vi "Tools_System Memory Status.vi"(8 "error in (no error)":errorcluster) -> (0 "error out":errorcluster, 1 "Free memory (%)":dbl, 2 "Free memory (MB)":dbl, 3 "Total memory (MB)":dbl)   [LabVIEW 2013]
uses:
  kernel32.dll
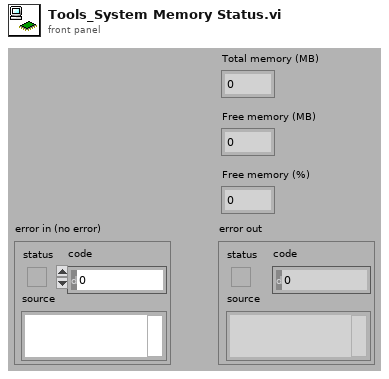
[diagram p1: front panel]
types:
  T1 = cluster{"dwLength":u32, "dwMemoryLoad":u32, "ullTotalPhys":u64, "ullAvailPhys":u64, "ullTotalPageFile":u64, "ullAvailPageFile":u64, "ullTotalVirtual":u64, "ullAvailVirtual":u64, "ullAvailExtendedVirtual":u64}
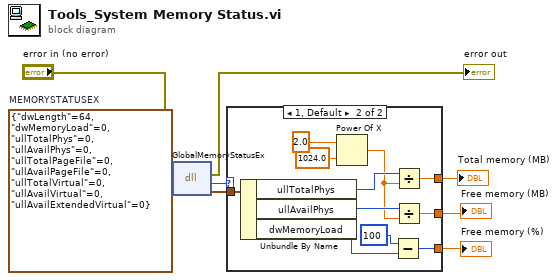
[diagram p0: block diagram]
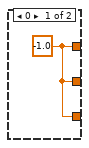
[diagram p2: hidden frame]
diagram:
  w3 = T1 {"dwLength"=64, "dwMemoryLoad"=0, "ullTotalPhys"=0, "ullAvailPhys"=0, "ullTotalPageFile"=0, "ullAvailPageFile"=0, "ullTotalVirtual"=0, "ullAvailVirtual"=0, "ullAvailExtendedVirtual"=0}  # MEMORYSTATUSEX
  n1 = dll-call lib="kernel32.dll" fn="GlobalMemoryStatusEx"(error in="error in (no error)", w3) -> (error out=→"error out":errorcluster, "return type"=w4:i32, w5:T1)  [unwired: 2 in, 1 out]
  n2 = case shown="1, Default" w4 {
    tunnel: w5 -> [_ w20]
    tunnel: [w9 w10] -> w8
    tunnel: [w9 w14] -> w6
    tunnel: [w9 w13] -> w7
    frame 0 {
      w9 = -1.0
    }
    frame 1, Default {
      n3 = Unbundle By Name(w20) -> ("ullTotalPhys"=w17:u64, "ullAvailPhys"=w16:u64, "dwMemoryLoad"=w11:u32)
      n4 = Power Of X(1:1024.0 ("x"), 2:2.0 ("y")) -> (0:w15:dbl)
      n5 = Subtract(x=u32 100, y=w11) -> (x-y=w10:u32)
      n6 = Divide(x=w17, y=w15) -> (x/y=w14:dbl)
      n7 = Divide(x=w16, y=w15) -> (x/y=w13:dbl)
    }
  }
  "Free memory (%)" <- w8
  "Free memory (MB)" <- w7
  "Total memory (MB)" <- w6
